vi "Set_Gain_DLPCA-200_Alex.vi"(3 "error in":errorcluster, 4 "Status":i32, 5 "Gain  [V/A]":T1(ring), 6 "index":i32) -> (0 "error out":errorcluster, 1 "Status_out":i32, 2 "index_out":i32)   [LabVIEW 2016, in "FEMTO_LUCI-10.lvlib"]
uses:
  LUCI-10/FEMTO_LUCI-10.lvlib
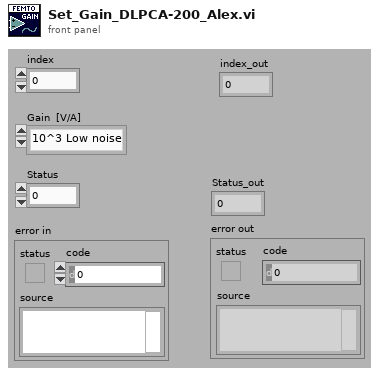
[diagram p1: front panel]
types:
  T1 = enum16{"10^3 Low noise", "10^4 Low noise", "10^5 Low noise", "10^6 Low noise", "10^7 Low noise", "10^8 Low noise", "10^9 Low noise", "10^10 High speed", "10^11 High speed"}
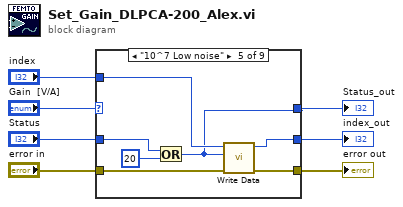
[diagram p0: block diagram]
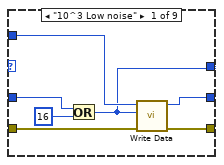
[diagram p2: hidden frame]
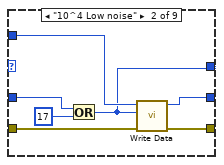
[diagram p3: hidden frame]
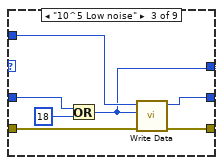
[diagram p4: hidden frame]
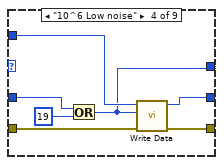
[diagram p5: hidden frame]
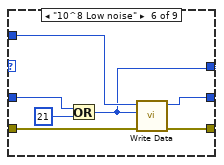
[diagram p6: hidden frame]
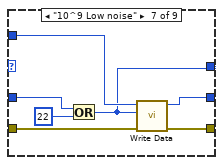
[diagram p7: hidden frame]
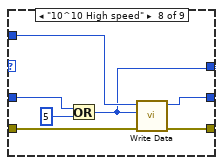
[diagram p8: hidden frame]
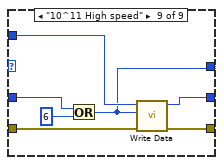
[diagram p9: hidden frame]
diagram:
  n1 = case shown="\"10^7 Low noise\"" "Gain  [V/A]" {
    tunnel: "index" -> [w14 w21 w28 w35 w42 w49 w56 w63 w70]
    tunnel: [w13 w20 w27 w34 w41 w48 w55 w62 w69] -> w4
    tunnel: "error in" -> [w12 w19 w26 w33 w40 w47 w54 w61 w68]
    tunnel: [w11 w18 w25 w32 w39 w46 w53 w60 w67] -> w6
    tunnel: "Status" -> [w9 w16 w23 w30 w37 w44 w51 w58 w65]
    tunnel: [w8 w15 w22 w29 w36 w43 w50 w57 w64] -> w1
    frame "10^3 Low noise" {
      n2 = Or(x=w9, y=16 ("data_low")) -> (x .or. y?=w8:i32)
      n3 = call "Write Data.vi"("error in (no error)"=w12, "data_low"=w8, "index"=w14) -> ("error out"=w11:errorcluster, "index_out"=w13:i32)  [unwired: 7 in]
    }
    frame "10^4 Low noise" {
      n4 = Or(x=w16, y=17 ("data_low")) -> (x .or. y?=w15:i32)
      n5 = call "Write Data.vi"("error in (no error)"=w19, "data_low"=w15, "index"=w21) -> ("error out"=w18:errorcluster, "index_out"=w20:i32)  [unwired: 7 in]
    }
    frame "10^5 Low noise" {
      n6 = Or(x=w23, y=18 ("data_low")) -> (x .or. y?=w22:i32)
      n7 = call "Write Data.vi"("error in (no error)"=w26, "data_low"=w22, "index"=w28) -> ("error out"=w25:errorcluster, "index_out"=w27:i32)  [unwired: 7 in]
    }
    frame "10^6 Low noise" {
      n8 = Or(x=w30, y=19 ("data_low")) -> (x .or. y?=w29:i32)
      n9 = call "Write Data.vi"("error in (no error)"=w33, "data_low"=w29, "index"=w35) -> ("error out"=w32:errorcluster, "index_out"=w34:i32)  [unwired: 7 in]
    }
    frame "10^7 Low noise" {
      n10 = Or(x=w37, y=20 ("data_low")) -> (x .or. y?=w36:i32)
      n11 = call "Write Data.vi"("error in (no error)"=w40, "data_low"=w36, "index"=w42) -> ("error out"=w39:errorcluster, "index_out"=w41:i32)  [unwired: 7 in]
    }
    frame "10^8 Low noise" {
      n12 = Or(x=w44, y=21 ("data_low")) -> (x .or. y?=w43:i32)
      n13 = call "Write Data.vi"("error in (no error)"=w47, "data_low"=w43, "index"=w49) -> ("error out"=w46:errorcluster, "index_out"=w48:i32)  [unwired: 7 in]
    }
    frame "10^9 Low noise" {
      n14 = Or(x=w51, y=22 ("data_low")) -> (x .or. y?=w50:i32)
      n15 = call "Write Data.vi"("error in (no error)"=w54, "data_low"=w50, "index"=w56) -> ("error out"=w53:errorcluster, "index_out"=w55:i32)  [unwired: 7 in]
    }
    frame "10^10 High speed" {
      n16 = Or(x=w58, y=5 ("data_low")) -> (x .or. y?=w57:i32)
      n17 = call "Write Data.vi"("error in (no error)"=w61, "data_low"=w57, "index"=w63) -> ("error out"=w60:errorcluster, "index_out"=w62:i32)  [unwired: 7 in]
    }
    frame "10^11 High speed" {
      n18 = Or(x=w65, y=6 ("data_low")) -> (x .or. y?=w64:i32)
      n19 = call "Write Data.vi"("error in (no error)"=w68, "data_low"=w64, "index"=w70) -> ("error out"=w67:errorcluster, "index_out"=w69:i32)  [unwired: 7 in]
    }
  }
  "index_out" <- w4
  "error out" <- w6
  "Status_out" <- w1
